vi "Approximately equals (1D DBL).vi"(7 "dy":dbl, 10 "y":dbl[](array[numeric]), 11 "x":dbl[](array[numeric])) -> (3 "x between (y-dy),(y+dy)?":bool)   [LabVIEW 2011, in "COSYLib.lvlib"]
doc: "Returns TRUE if all x[i] fall within the range (y[i]-dy, y[i]+dy)."
uses:
  COSYLib.lvlib
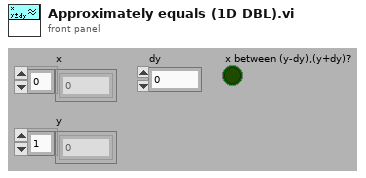
[diagram p1: front panel]
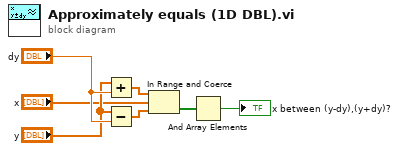
[diagram p0: block diagram]
diagram:
  n1 = Add(x="y", y="dy") -> (x+y=w6:dbl[])
  n2 = Subtract(x="y", y="dy") -> (x-y=w7:dbl[])
  n3 = In Range and Coerce(upper limit=w6, x="x", lower limit=w7) -> (In Range?=w2:bool[])  [unwired: 1 out]
  n4 = And Array Elements(Boolean array=w2) -> (logical AND=→"x between (y-dy),(y+dy)?":bool)
